vi "Test001.vi"() -> ()   [LabVIEW 2018]
uses:
  <vilib>/vision/NI_Vision_Development_Module.lvlib
panel:
  out "error out":errorcluster
  out "Image":T1(plugin-control)
  out "G 2":T1(plugin-control)
  out "G":T1(plugin-control)
  out "R":T1(plugin-control)
  out "Show_01 4":T1(plugin-control)
  out "Show_01 3":T1(plugin-control)
  out "error out 2":errorcluster
  in  "File Path 2":path=path "D:/Life/20191001_Accordance/Project/EPISIL/20200806-Camera/20200716/getimg_003.bmp"
  out "Show_01 2":T1(plugin-control)
  out "Show_01":T1(plugin-control)
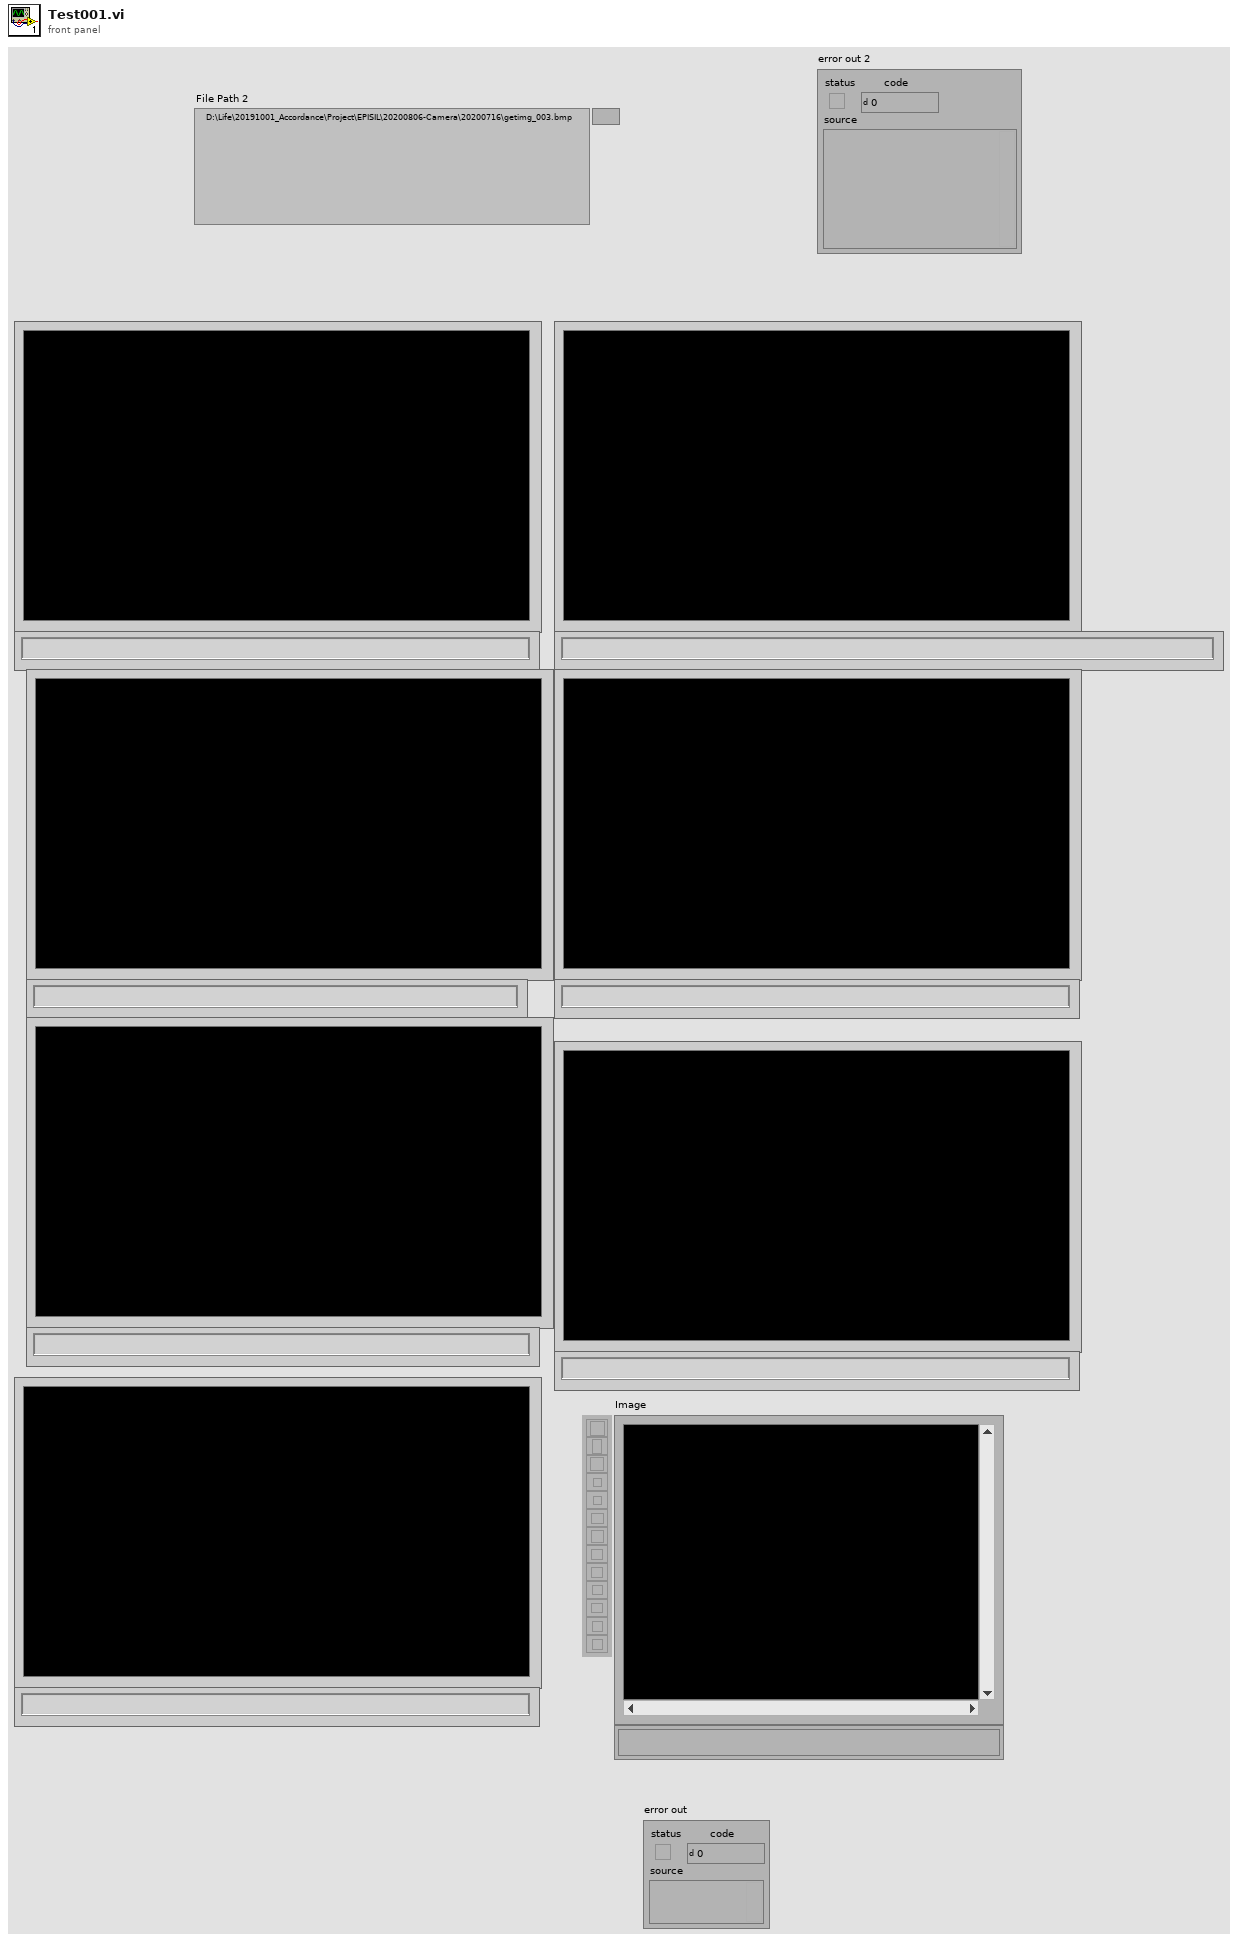
[diagram p1: front panel]
types:
  T1 = typedef "IMAQ Image.ctl" = refnum<image>
  T2 = typedef "Image Type" = u32
  T3 = typedef "IMAQ Rectangle" = cluster{"Left":i32, "Top":i32, "Right":i32, "Bottom":i32, "Rotation":dbl}
  T4 = cluster{"Left":i32, "Top":i32, "Right":i32, "Bottom":i32}
  T5 = typedef "ROI Descriptor" = cluster{"Global Rectangle":i32[], "Contours":cluster{"ID":enum32{"External", "Internal"}, "Type":u32, "Coordinates":i32[]}[]}
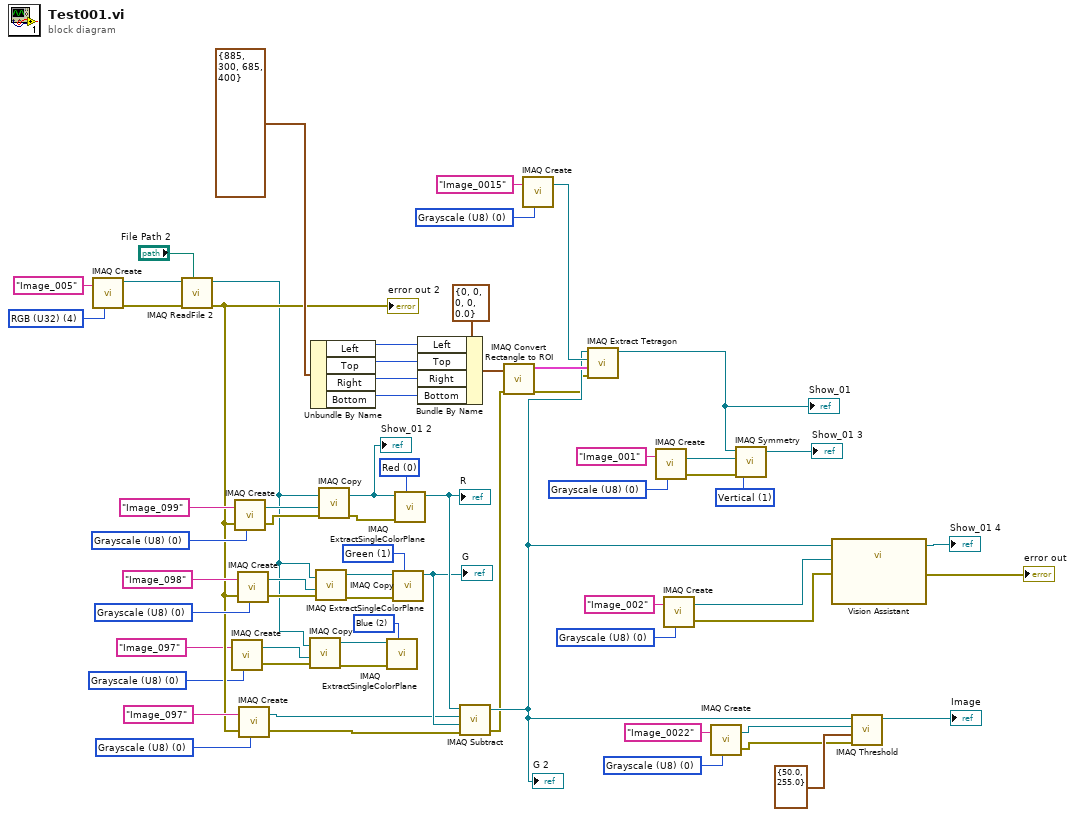
[diagram p0: block diagram]
diagram:
  w2 = 2 items=["Red", "Green", "Blue", "Hue", "Saturation", "Luminance", "Value", "Intensity"] ("Color Plane")
  w4 = T2 0 items=["Grayscale (U8)", "Grayscale (I16)", "Grayscale (SGL)", "Complex (CSG)", "RGB (U32)", "HSL (U32)", "RGB (U64)", "Grayscale (U16)"] ("Image Type")
  w20 = T2 0 items=["Grayscale (U8)", "Grayscale (I16)", "Grayscale (SGL)", "Complex (CSG)", "RGB (U32)", "HSL (U32)", "RGB (U64)", "Grayscale (U16)"] ("Image Type")
  w28 = u32 1 items=["Horizontal", "Vertical", "Central", "1st Diagonal", "2nd Diagonal"] ("Type of Symmetry")
  w31 = T2 0 items=["Grayscale (U8)", "Grayscale (I16)", "Grayscale (SGL)", "Complex (CSG)", "RGB (U32)", "HSL (U32)", "RGB (U64)", "Grayscale (U16)"] ("Image Type")
  w35 = T2 0 items=["Grayscale (U8)", "Grayscale (I16)", "Grayscale (SGL)", "Complex (CSG)", "RGB (U32)", "HSL (U32)", "RGB (U64)", "Grayscale (U16)"] ("Image Type")
  w41 = 1 items=["Red", "Green", "Blue", "Hue", "Saturation", "Luminance", "Value", "Intensity"] ("Color Plane")
  w43 = 0 items=["Red", "Green", "Blue", "Hue", "Saturation", "Luminance", "Value", "Intensity"] ("Color Plane")
  w46 = T2 0 items=["Grayscale (U8)", "Grayscale (I16)", "Grayscale (SGL)", "Complex (CSG)", "RGB (U32)", "HSL (U32)", "RGB (U64)", "Grayscale (U16)"] ("Image Type")
  w48 = T2 0 items=["Grayscale (U8)", "Grayscale (I16)", "Grayscale (SGL)", "Complex (CSG)", "RGB (U32)", "HSL (U32)", "RGB (U64)", "Grayscale (U16)"] ("Image Type")
  w51 = T2 0 items=["Grayscale (U8)", "Grayscale (I16)", "Grayscale (SGL)", "Complex (CSG)", "RGB (U32)", "HSL (U32)", "RGB (U64)", "Grayscale (U16)"] ("Image Type")
  w54 = T2 0 items=["Grayscale (U8)", "Grayscale (I16)", "Grayscale (SGL)", "Complex (CSG)", "RGB (U32)", "HSL (U32)", "RGB (U64)", "Grayscale (U16)"] ("Image Type")
  w66 = T2 4 items=["Grayscale (U8)", "Grayscale (I16)", "Grayscale (SGL)", "Complex (CSG)", "RGB (U32)", "HSL (U32)", "RGB (U64)", "Grayscale (U16)"] ("Image Type")
  n1 = call "IMAQ Create"("Image Name"="Image_005", "Image Type"=w66) -> ("New Image"=w65:T1, "error out"=w64:errorcluster)  [unwired: 3 in]
  n2 = call "IMAQ ReadFile 2"("File Path"="File Path 2", "error in (no error)"=w64, "Image"=w65) -> ("error out"=w16:errorcluster, "Image Out"=w3:T1)  [unwired: 4 in, 3 out]
  "error out 2" <- w16
  n3 = call "IMAQ Create"("Image Name"="Image_097", "Image Type"=w4) -> ("New Image"=w6:T1, "error out"=w9:errorcluster)  [unwired: 3 in]
  n4 = call "IMAQ Create"("Image Name"="Image_099", "Image Type"=w48, "error in (no error)"=w16) -> ("New Image"=w47:T1, "error out"=w14:errorcluster)  [unwired: 2 in]
  n5 = call "IMAQ Create"("Image Name"="Image_098", "Image Type"=w46, "error in (no error)"=w16) -> ("New Image"=w44:T1, "error out"=w15:errorcluster)  [unwired: 2 in]
  n6 = call "IMAQ Create"("Image Name"="Image_097", "Image Type"=w35, "error in (no error)"=w16) -> ("New Image"=w34:T1, "error out"=w33:errorcluster)  [unwired: 2 in]
  n7 = call "IMAQ Copy"("error in (no error)"=w9, "Image Dst"=w6, "Image Src"=w3) -> ("error out"=w8:errorcluster, "Image Dst Out"=w7:T1)  [unwired: 3 in]
  n8 = Unbundle By Name(T4 {"Left"=885, "Top"=300, "Right"=685, "Bottom"=400} ("Rectangle")) -> ("Left"=w60:i32, "Top"=w59:i32, "Right"=w58:i32, "Bottom"=w57:i32)
  n9 = call "IMAQ Copy"("error in (no error)"=w15, "Image Dst"=w44, "Image Src"=w3) -> ("error out"=w39:errorcluster, "Image Dst Out"=w42:T1)  [unwired: 3 in]
  n10 = call "IMAQ Copy"("error in (no error)"=w14, "Image Dst"=w47, "Image Src"=w3) -> ("error out"=w40:errorcluster, "Image Dst Out"=w1:T1)  [unwired: 3 in]
  "Show_01 2" <- w1
  n11 = call "IMAQ ExtractSingleColorPlane"("Color Plane"=w2, "error in (no error)"=w8, "Image Src"=w7) -> ()  [unwired: 7 in, 2 out]
  n12 = call "IMAQ ExtractSingleColorPlane"("Color Plane"=w41, "error in (no error)"=w39, "Image Src"=w42) -> ("Image Dst Out"=w37:T1)  [unwired: 7 in, 1 out]
  "G" <- w37
  n13 = call "IMAQ ExtractSingleColorPlane"("Color Plane"=w43, "error in (no error)"=w40, "Image Src"=w1) -> ("Image Dst Out"=w38:T1)  [unwired: 7 in, 1 out]
  "R" <- w38
  n14 = Bundle By Name(cluster=T3 {"Left"=0, "Top"=0, "Right"=0, "Bottom"=0, "Rotation"=0.0} ("Rectangle"), "Left"=w60, "Top"=w59, "Right"=w58, "Bottom"=w57) -> (w56:T3)
  n15 = call "IMAQ Subtract"("Image Src A"=w38, "Image Dst"=w34, "Image Src B"=w37, "error in (no error)"=w33) -> ("Image Dst Out"=w17:T1, "error out"=w13:errorcluster)  [unwired: 3 in]
  "G 2" <- w17
  n16 = call "IMAQ Convert Rectangle to ROI"("error in (no error)"=w13, "Rectangle"=w56) -> ("error out"=w12:errorcluster, "ROI Descriptor"=w55:T5)  [unwired: 7 in]
  n17 = call "IMAQ Create"("Image Name"="Image_0015", "Image Type"=w54) -> ("New Image"=w52:T1)  [unwired: 3 in, 1 out]
  n18 = call-poly "IMAQ Extract Tetragon"("error in (no error)"=w12, "ROI Descriptor"=w55, "Image Dst"=w52, "Image Src"=w17) -> ("Image Dst Out"=w27:T1)  [unwired: 6 in, 1 out]
  "Show_01" <- w27
  n19 = call "IMAQ Create"("Image Name"="Image_001", "Image Type"=w31) -> ("New Image"=w30:T1, "error out"=w29:errorcluster)  [unwired: 3 in]
  n20 = call "IMAQ Create"("Image Name"="Image_002", "Image Type"=w51) -> ("New Image"=w26:T1, "error out"=w25:errorcluster)  [unwired: 3 in]
  n21 = call "IMAQ Create"("Image Name"="Image_0022", "Image Type"=w20) -> ("New Image"=w19:T1, "error out"=w11:errorcluster)  [unwired: 3 in]
  n22 = call "IMAQ Symmetry"("error in (no error)"=w29, "Type of Symmetry"=w28, "Image Dst"=w30, "Image Src"=w27) -> ("Image Dst Out"=→"Show_01 3":T1)  [unwired: 1 in, 1 out]
  n23 = call "Vision Assistant"("Image In"=w17, "Image Dst"=w26, "error in"=w25) -> ("Image Out"=→"Show_01 4":T1, "error out"=→"error out":errorcluster)  [unwired: 23 in]
  n24 = call "IMAQ Threshold"("error in (no error)"=w11, "Range"=cluster{"Lower value":sgl, "Upper value":sgl} {"Lower value"=50.0, "Upper value"=255.0}, "Image Dst"=w19, "Image Src"=w17) -> ("Image Dst Out"=→"Image":T1)  [unwired: 6 in, 1 out]
